vi "Generate Ao_ReadRPM AC Test V2.vi"(0 "Device Name":string="Dev1", 2 "rate":dbl=10000.0, 3 "frequency":dbl=62.5, 8 "offset":dbl=3.75, 9 "SquareWave duty cycle (%)":dbl=50.0, 10 "#Samples":i32=30000, 11 "amplitude (pk)":dbl=1.25) -> (15 "Ch1 Result":dbl=nan, 16 "Ch2 Result":dbl=nan, 19 "error out":errorcluster)   [LabVIEW 2015]
uses:
  <vilib>/DAQmx/write.llb/DAQmx Write (Analog 1D Wfm NChan NSamp).vi
  <vilib>/DAQmx/create/channels.llb/DAQmx Create Channel (AO-Voltage-Basic).vi
  <vilib>/DAQmx/configure/timing.llb/DAQmx Timing (Sample Clock).vi
  <vilib>/DAQmx/miscellaneous.llb/DAQmx Fill In Error Info.vi
  <resource>/objmgr/daqmx.rc
  <vilib>/measure/NI_MABase.lvlib
panel:
  out "Waveform Graph":waveform(dbl)(graph)={"t0"=timestamp(0 s since 1904-01-01), "dt"=0.0001, "Y"=array[30000 elements]}
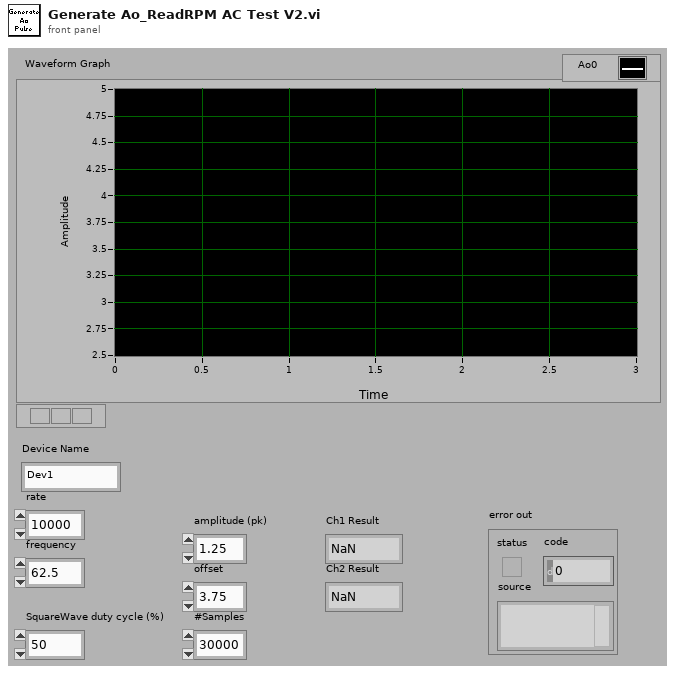
[diagram p1: front panel]
types:
  T1 = enum16{"Sine Wave", "Triangle Wave", "Square Wave", "Sawtooth Wave"}
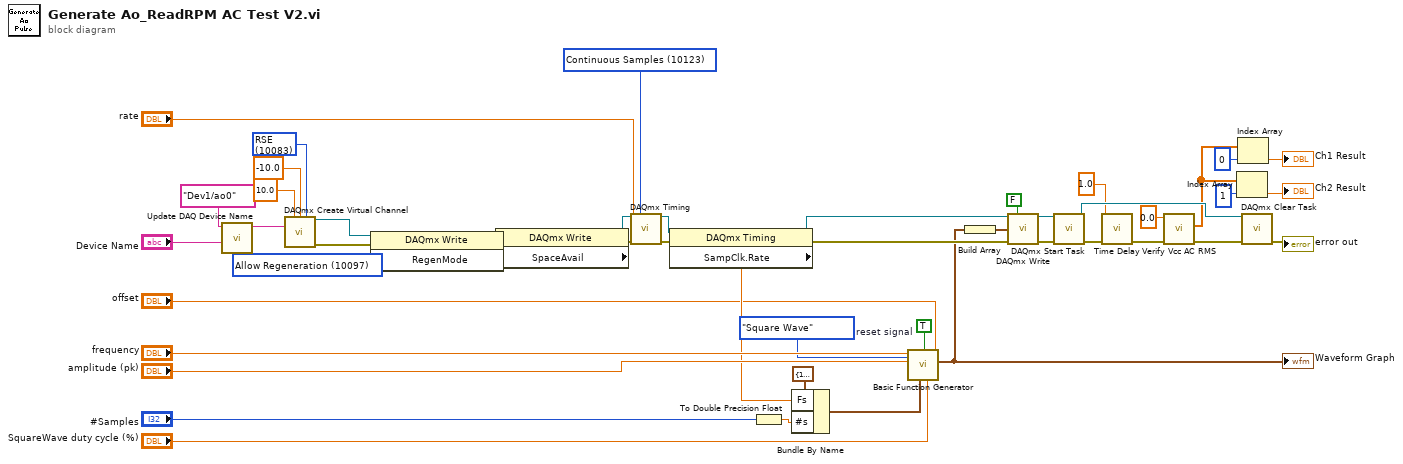
[diagram p0: block diagram]
diagram:
  w15 = 10123 items=["Finite Samples"=10178, "Continuous Samples"=10123, "Hardware Timed Single Point"=12522] ("sample mode")
  w18 = 10083 items=["Default"=-1, "RSE"=10083, "Differential"=10106, "Pseudodifferential"=12529] ("output terminal configuration")
  w30 = TRUE  # reset signal
  w45 = 10097 items=["Allow Regeneration"=10097, "Do Not Allow Regeneration"=10158] ("RegenMode")
  n1 = call "Update DAQ Device Name.vi"("Device Name"="Device Name", "Lines in (String)"="Dev1/ao0" ("Channel names 2")) -> ("Lines out (DAQmx Physical Channels)"=w8:tag)  [unwired: 9 in]
  n2 = call-poly <vilib>:"DAQmx Create Virtual Channel.vi"("maximum value"=10.0, "minimum value"=-10.0, "output terminal configuration"=w18, "physical channels"=w8) -> ("task out"=w47:refnum<k21>, "error out"=w46:errorcluster)  [unwired: 10 in]
  n3 = property class="DAQmx Write"(reference=w47, error in=w46, "RegenMode"=w45) -> (reference out=w43:refnum<k21>, error out=w44:errorcluster)
  n4 = property class="DAQmx Write" props=["SpaceAvail"](reference=w43, error in=w44) -> (reference out=w42:refnum<k21>, error out=w41:errorcluster)  [unwired: 1 out]
  n5 = call-poly <vilib>:"DAQmx Timing.vi"("task/channels in"=w42, "sample mode"=w15, "rate"="rate", "error in"=w41) -> ("task out"=w40:refnum<k21>, "error out"=w39:errorcluster)  [unwired: 10 in]
  n6 = property class="DAQmx Timing"(reference=w40, error in=w39) -> (reference out=w23:refnum<k21>, error out=w24:errorcluster, "SampClk.Rate"=w33:dbl)
  n7 = To Double Precision Float(number="#Samples") -> (double precision float=w32:dbl)
  n8 = Bundle By Name(cluster=cluster{"Fs":dbl, "#s":dbl} {"Fs"=1000.0, "#s"=1000.0} ("sampling info"), "Fs"=w33, "#s"=w32) -> (w35:cluster{"Fs":dbl, "#s":dbl})
  n9 = call <vilib>:"Basic Function Generator.vi"("offset"="offset", "square wave duty cycle (%)"="SquareWave duty cycle (%)", "reset signal"=w30, "sampling info"=w35, "signal type"=T1."Square Wave", "amplitude"="amplitude (pk)", "frequency"="frequency") -> ("signal out"=w16:waveform(dbl))  [unwired: 2 in, 2 out]
  "Waveform Graph" <- w16
  n10 = Build Array(w16) -> (w17:waveform(dbl)[])
  n11 = call-poly <vilib>:"DAQmx Write.vi"("task/channels in"=w23, "auto start"=FALSE, "data"=w17, "error in"=w24) -> ("task out"=w21:refnum<k21>, "error out"=w22:errorcluster)  [unwired: 9 in, 1 out]
  n12 = call <vilib>:"DAQmx Start Task.vi"("task/channels in"=w21, "error in"=w22) -> ("task out"=w13:refnum<k21>, "error out"=w12:errorcluster)  [unwired: 12 in]
  n13 = call "Time Delay"("error in (no error)"=w12, "Delay Time (s)"=1.0) -> ("error out"=w11:errorcluster)  [unwired: 9 in]
  n14 = call "Verify Vcc AC RMS.vi"("error in"=w11, "Delay Time (s)"=0.0) -> ("error out"=w14:errorcluster, "Ch Values"=w5:dbl[])  [unwired: 7 in, 1 out]
  n15 = Index Array(array=w5, index=1) -> (element=→"Ch2 Result":dbl)
  n16 = Index Array(array=w5, index=0) -> (element=→"Ch1 Result":dbl)
  n17 = call <vilib>:"DAQmx Clear Task.vi"("task in"=w13, "error in"=w14) -> ("error out"=→"error out":errorcluster)  [unwired: 13 in]
